vi "Paths and Data to Map.vi"(7 "map in":map{string, map{string, string[]}}(c390), 8 "error in":errorcluster, 9 "Data":variant, 10 "Paths":variant) -> (0 "error out":errorcluster, 2 "map out":map{string, map{string, string[]}}(c390)={"llab_060"={"v000"=["$$X$$"], "v006"=["$$X$$"]}, "llab_061"={"d000"=["0"], "v000"=["$$X$$"], "v003"=["$$X$$"], "v006"=["$$X$$"]}, "llab_063"={"d001"=["5"]}}, 4 "paths":string[](array[string]))   [LabVIEW 2019, in "LV-Data.PGSQL.lvclass"]
uses:
  LV-Data.PGSQL.lvclass
  Typedefs/Errors--enum.ctl
  <vilib>/Utility/miscctls.llb/LVMapReplaceAction.ctl
  <vilib>/Utility/Data Type/NI_Data Type.lvlib
  8e915fe2-c280-4114-bdfd-b6e2c6cb9e36.vi
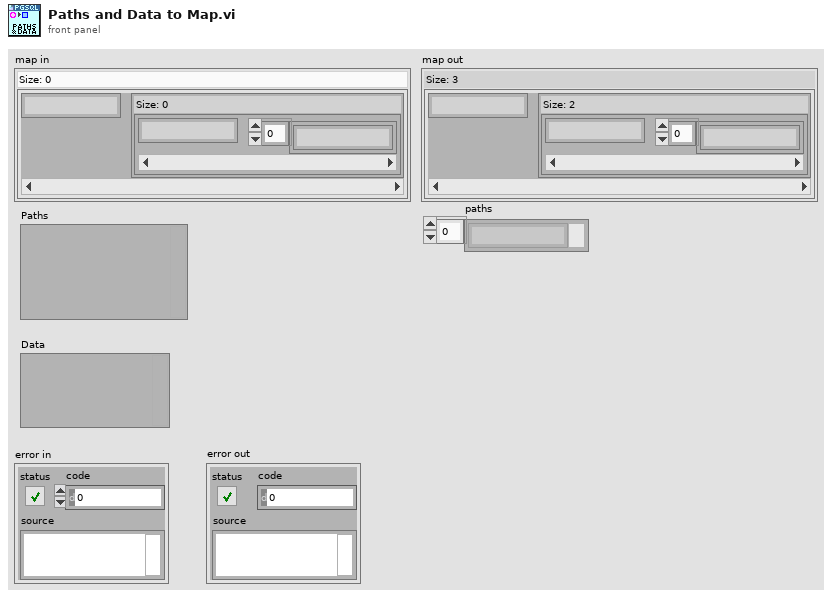
[diagram p1: front panel]
types:
  T1 = typedef "NI_Data Type.lvlib/Data Type.ctl" = enum8{"Invalid Type", "Void", "I8", "I16", "I32", "I64", "U8", "U16", "U32", "U64", "Single Float", "Double Float", "Extended Float", "Single Complex", "Double Complex", "Extended Complex", "Enum U8", "Enum U16", "Enum U32", "Enum U64", "Single Float With Unit", "Double Float With Unit", "Extended Float With Unit", "Single Complex with Unit", "Double Complex with Unit", "Extended Complex with Unit", "Boolean", "String", "Path", "Picture", "Tag", "Array", "Cluster", "Variant", "LV Variant", "Waveform", "Timestamp", "Digital Waveform", "Digital Data", "ExpressData", "Refnum", "External Data", "VI", "Poly VI", "LabVIEW Class Instance", "Fixed Point", "Set Collection", "Map Collection"}
  T2 = typedef "LV-Data.PGSQL.lvclass/Errors--enum.ctl" = enum16{"0: None", "5005: Path Type Not Supported", "5006: Number of Variables", "5007: Number of data points", "5008: Cannot write two data points", "5030: Start and End Times Identical", "5031: Input is not wholly", "5032: Undefined Timestamps", "5033: Bad path or paths", "5040: Invalid Instrument Name", "5050: Column can only hold string", "5051: Column can only hold bool", "5052: Column can only hold double", "5053: Column can only hold int"}
  T3 = typedef "LVMapReplaceAction.ctl" = enum32{"Modify Entry only if found", "Add or Modify Entry", "Delete Entry"}
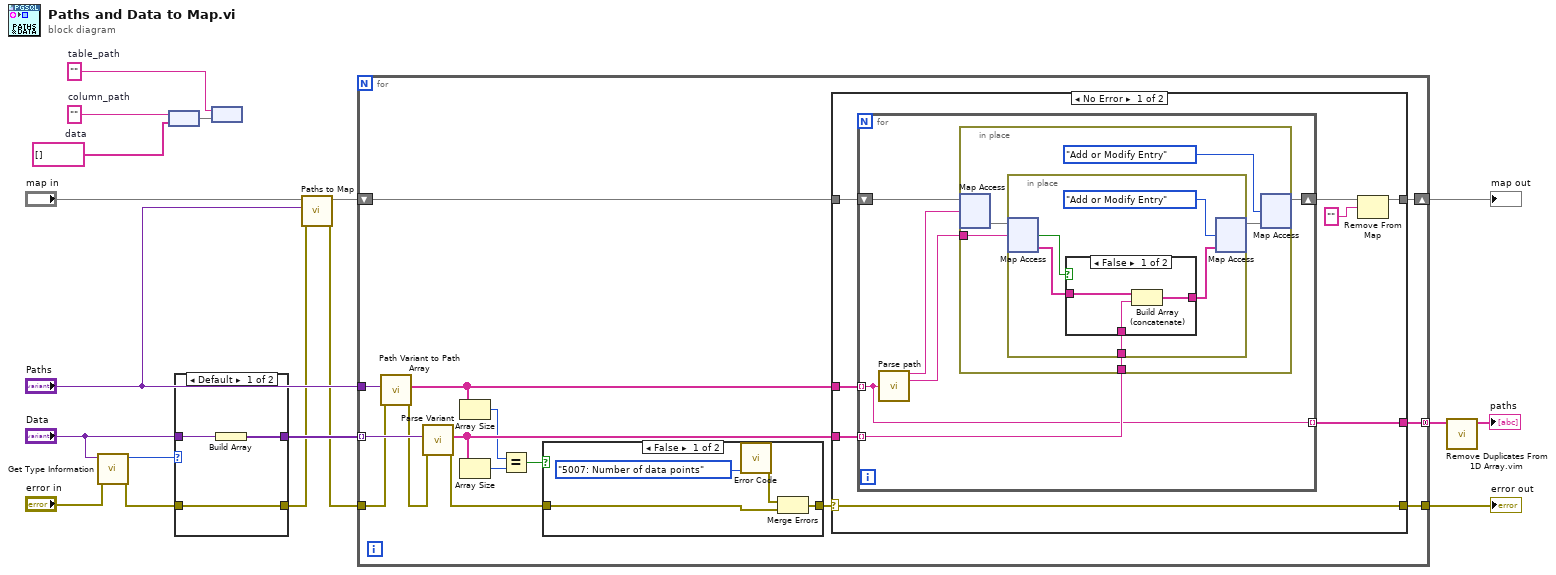
[diagram p0: block diagram]
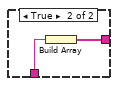
[diagram p3: hidden frame]
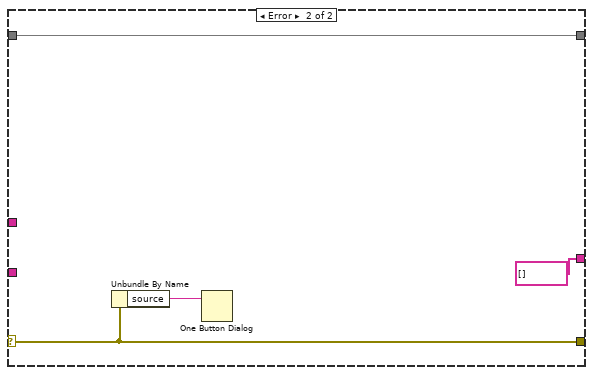
[diagram p4: hidden frame]
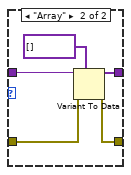
[diagram p5: hidden frame]
diagram:
  w5 = string[] []  # data
  w6 = ""  # column_path
  w4 = ""  # table_path
  n1 = call <vilib>:"Get Type Information.vi"("error in (no error)"="error in", "variant"="Data") -> ("error out"=w8:errorcluster, "type"=w10:T1)  [unwired: 5 in, 3 out]
  n2 = node(w6, w5) -> (w7:map{string, string[]})
  n3 = case shown="Default" w10 {
    tunnel: [w20 w25] -> w17
    tunnel: w8 -> [w19 w24]
    tunnel: [w19 w23] -> w13
    tunnel: "Data" -> [w21 w22]
    frame Default {
      n4 = Build Array(w21) -> (w20:variant[])
    }
    frame "Array" {
      n5 = Variant To Data(error in=w24, type=variant[] [], Variant=w22) -> (data=w25:variant[], error out=w23:errorcluster)
    }
  }
  n6 = node(w4, w7) -> ()  [unwired: 1 out]
  n7 = call "Paths to Map.vi"("error in"=w13, "Paths"="Paths", "map in"="map in") -> ("error out"=w12:errorcluster, "map out"=w15:map{string, map{string, string[]}})  [unwired: 7 in]
  n8 = for {
    tunnel: w17 -> [w41] mode=indexing
    tunnel: "Paths" -> [w35]
    tunnel: w12 -> [w36]
    tunnel: [w38] -> w18
    shift-right: [w40] -> w3
    shift-left: w15 -> [w37]
    tunnel: [w34] -> w2 mode=concatenating
    n9 = call "Path Variant to Path Array.vi"("error in"=w36, "Paths"=w35) -> ("error out"=w39:errorcluster, "Paths"=w33:string[])  [unwired: 8 in]
    n10 = call "Parse Variant.vi"("error in"=w39, "Data"=w41) -> ("error out"=w28:errorcluster, "Data"=w32:string[])  [unwired: 5 in, 3 out]
    n11 = Array Size(array=w33) -> (size(s)=w30:i32)
    n12 = Array Size(array=w32) -> (size(s)=w31:i32)
    n13 = Equal?(x=w30, y=w31) -> (x = y?=w27:bool)
    n14 = case shown="False" w27 {
      tunnel: [w43 w46] -> w29
      tunnel: w28 -> [w42 w46]
      frame False {
        n15 = call "Error Code.vi"("Error code"=Errors--enum."5007: Number of data points") -> ("error out"=w44:errorcluster)  [unwired: 10 in]
        n16 = Merge Errors(w44, w42) -> (w43:errorcluster)
      }
      frame True {
      }
    }
    n17 = case shown="No Error" w29 {
      selector: w29 -> [w48 w78]
      tunnel: w37 -> [w54 w79]
      tunnel: w32 -> [w53 _]
      tunnel: [w50 w79] -> w40
      tunnel: w33 -> [w49 _]
      tunnel: [w48 w78] -> w38
      tunnel: [w47 string[] []] -> w34
      frame No Error {
        n18 = for {
          tunnel: w49 -> [w55] mode=indexing
          shift-right: [w57] -> w52
          shift-left: w54 -> [w60]
          tunnel: w53 -> [w56] mode=indexing
          tunnel: [w55] -> w47 mode=indexing
          n19 = call "Parse path.vi"("PG Path"=w55) -> ("Table path"=w59:string, "Column path"=w58:string)  [unwired: 10 in, 3 out]
          n20 = in-place {
            in-place-border: w58 -> [w64]
            in-place-border: w56 -> [w61]
            n21 = in-place-map #1(w60, w59) -> (w65:map{string, string[]})  [unwired: 1 in, 1 out]
            n22 = in-place {
              in-place-border: w61 -> [w68]
              n23 = in-place-map #2(w65, w64) -> (w66:string[], w69:bool)  [unwired: 1 in]
              n24 = case shown="False" w69 {
                tunnel: w68 -> [w72 w74]
                tunnel: [w71 w75] -> w67
                tunnel: w66 -> [w73 _]
                frame False {
                  n25 = Build Array (concatenate)(w73, w72) -> (w71:string[])
                }
                frame True {
                  n26 = Build Array(w74) -> (w75:string[])
                }
              }
              n27 = in-place-map #2(w67, LVMapReplaceAction."Add or Modify Entry" ("action")) -> (w63:map{string, string[]})  [unwired: 2 out]
            }
            n28 = in-place-map #1(w63, LVMapReplaceAction."Add or Modify Entry" ("action")) -> (w57:map{string, map{string, string[]}})  [unwired: 2 out]
          }
        }
        n29 = Remove From Map(10:"" ("key"), 11:w52) -> (3:w50:map{string, map{string, string[]}})  [unwired: 2 out]
      }
      frame Error {
        n30 = Unbundle By Name(w78) -> ("source"=w77:string)
        n31 = One Button Dialog(message=w77) -> ()  [unwired: 1 in, 1 out]
      }
    }
  }
  "error out" <- w18
  "map out" <- w3
  n32 = call "Remove Duplicates From 1D Array.vim"("array"=w2) -> ("array with duplicates removed"=→"paths":string[])  [unwired: 10 in]
